vi "myRIO v1.0 Reserve Channel.vi"(5 "Allow multiple opens?":bool, 7 "Owner":string, 8 "error in (no error)":errorcluster, 9 "Mutex ID":i32, 10 "Connector":T1=enum."ConnectorA", 11 "Channel Name":string) -> (0 "error out":errorcluster)   [LabVIEW 2021]
uses:
  <vilib>/myRIO/Common/Instrument Driver Framework/myRIO v1.0/Resource Manager/typedefs/myRIO v1.0 Connector List.ctl
  <vilib>/myRIO/Common/Instrument Driver Framework/Utilities/typedefs/Resource Manager Action Enum.ctl
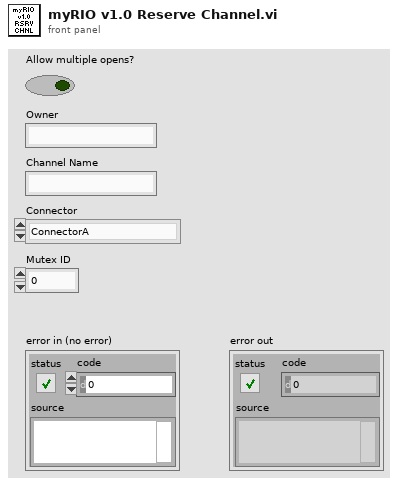
[diagram p1: front panel]
types:
  T1 = typedef "myRIO v1.0 Connector List.ctl" = enum32{"None", "ConnectorA", "ConnectorB", "ConnectorC"}
  T2 = typedef "Resource Manager Action Enum.ctl" = enum16{"Lock", "Unlock"}
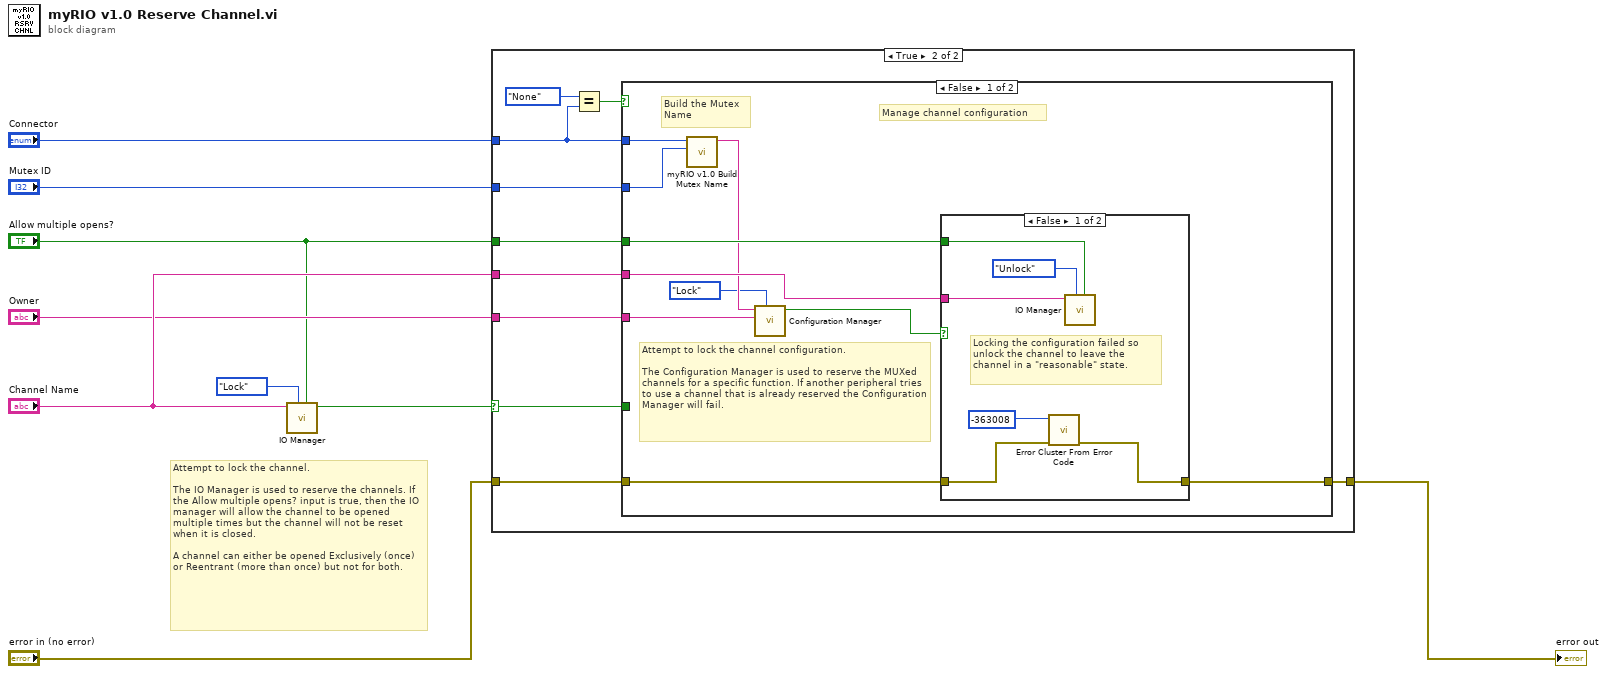
[diagram p0: block diagram]
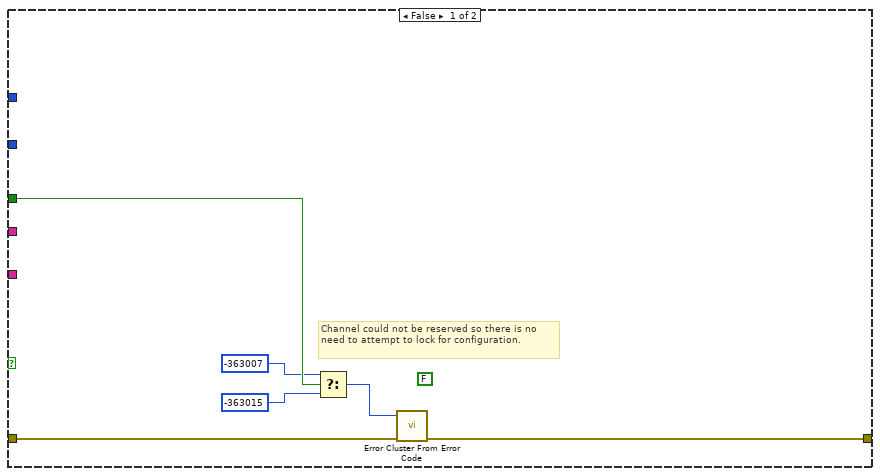
[diagram p2: hidden frame]
diagram:
  # "Attempt to lock the channel.\n\nThe IO Manager is used to reserve the channels. If the Allow multiple opens? input is true, then the IO manager will allow the channel to be opened multiple times but the channel will not be reset when it is closed.\n\nA channel can either be opened Exclusively (once) or Reentrant (more than once) but not for both."
  n1 = call <vilib>:"IO Manager.vi"("Reentrant?"="Allow multiple opens?", "Actions"=Resource_Manager_Action_Enum."Lock", "Mutex Name"="Channel Name") -> ("Success?"=w2:bool)  [unwired: 8 in]
  n2 = case shown="True" w2 {
    selector: w2 -> [_ w18]
    tunnel: "Channel Name" -> [_ w25]
    tunnel: "Owner" -> [_ w24]
    tunnel: "Allow multiple opens?" -> [w13 w23]
    tunnel: "Mutex ID" -> [_ w22]
    tunnel: "Connector" -> [_ w21]
    tunnel: "error in (no error)" -> [w15 w17]
    tunnel: [w14 w16] -> w3
    frame False {
      (unwired) FALSE ("Reentrant?")
      # "Channel could not be reserved so there is no need to attempt to lock for configuration."
      n3 = Select(t=-363007 ("error code (0)"), s=w13, f=-363015 ("error code (0)")) -> (s? t:f=w11:i32)
      n4 = call <vilib>:"Error Cluster From Error Code.vi"("error in (no error)"=w15, "error code (0)"=w11) -> ("error out"=w14:errorcluster)  [unwired: 7 in]
    }
    frame True {
      n5 = Equal?(x=myRIO_v1.0_Connector_List."None", y=w21) -> (x = y?=w19:bool)
      n6 = case shown="False" w19 {
        tunnel: w25 -> [w35 _]
        tunnel: w24 -> [w34 _]
        tunnel: w18 -> [_ _]
        tunnel: w23 -> [w33 _]
        tunnel: w21 -> [w32 _]
        tunnel: w22 -> [w31 _]
        tunnel: w17 -> [w27 w43]
        tunnel: [w26 w43] -> w16
        frame False {
          # "Attempt to lock the channel configuration.\n\nThe Configuration Manager is used to reserve the MUXed channels for a specific function. If another peripheral tries to use a channel that is already reserved the Configuration Manager will fail."
          # "Build the Mutex Name"
          # "Manage channel configuration"
          n7 = call <vilib>:"myRIO v1.0 Build Mutex Name.vi"("Mutex ID"=w31, "Connector"=w32) -> ("Mutex Name"=w30:string)  [unwired: 9 in]
          n8 = call <vilib>:"Configuration Manager.vi"("Actions"=Resource_Manager_Action_Enum."Lock", "Owner"=w34, "Mutex Name"=w30) -> ("Success?"=w28:bool)  [unwired: 8 in]
          n9 = case shown="False" w28 {
            tunnel: w35 -> [w40 _]
            tunnel: w33 -> [w39 _]
            tunnel: w27 -> [w38 w42]
            tunnel: [w36 w42] -> w26
            frame False {
              # "Locking the configuration failed so unlock the channel to leave the channel in a \"reasonable\" state."
              n10 = call <vilib>:"Error Cluster From Error Code.vi"("error in (no error)"=w38, "error code (0)"=-363008) -> ("error out"=w36:errorcluster)  [unwired: 7 in]
              n11 = call <vilib>:"IO Manager.vi"("Reentrant?"=w39, "Actions"=Resource_Manager_Action_Enum."Unlock", "Mutex Name"=w40) -> ()  [unwired: 8 in, 1 out]
            }
            frame True {
            }
          }
        }
        frame True {
          # "If there is no connector then there is no channel configuration to manage."
        }
      }
    }
  }
  "error out" <- w3
